vi "Calinski_Harabasz_Score.vi"(8 "error in (no error)":errorcluster caption="entrée d'erreur (pas d'erreur)", 10 "labels":string[][](array[string]), 11 "X":string[][](array[string])) -> (0 "error out":errorcluster caption="sortie d'erreur", 3 "Score":string)   [LabVIEW 2020]
doc: "Compute the Calinski and Harabasz score.\n\nIt is also known as the Variance Ratio Criterion.\n\nThe score is defined as ratio between the within-cluster dispersion and the between-cluster dispersion.\n\n\n\nParameters : \n\n- X : array-like, shape (n_samples, n_features)\nList of n_features-dimensional data points. Each row corresponds to a single data point.\n\n- labels : array-like, shape (n_samples,)\nPredicted labels for each sample.\n\nReturns : \n\n- score : float\nThe resulting Calinski-Harabasz score."
uses:
  Calinski_Harabasz_Score.lvclass
panel:
  out "Calinski_Harabasz_Score.lvclass":refnum<class "Calinski_Harabasz_Score.lvclass">
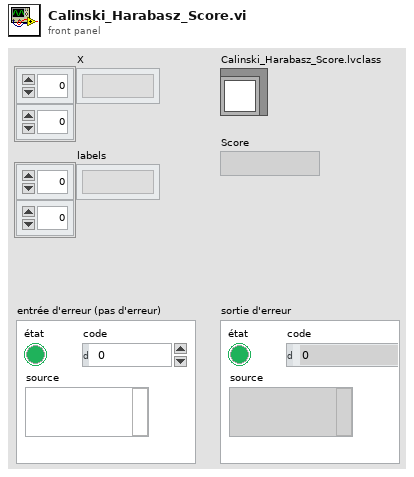
[diagram p1: front panel]
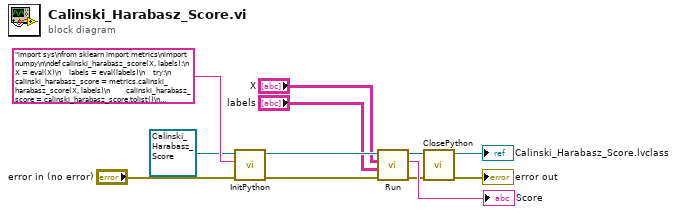
[diagram p0: block diagram]
diagram:
  n1 = call-dynamic "InitPython.vi"("error in (no error)"="error in (no error)", "Python Instruction"="import sys\nfrom sklearn import metrics\nimport numpy\n\ndef calinski_harabasz_score(X, labels):\n    X = eval(X)\n    labels = eval(labels)\n    try:\n        calinski_harabasz_score = metrics.calinski_harabasz_score(X, labels)\n        calinski_harabasz_score = calinski_harabasz_score.tolist()\n        return str(calinski_harabasz_score)\n    except:\n        erreur = sys.exc_info()\n        typerr = u\"%s\" % (erreur[0])\n        typerr = typerr[typerr.find(\"'\")+1:typerr.rfind(\"'\")]\n        msgerr = u\"%s\" % (erreur[1])\n        message = str('/!\\\\ {0} : {1}'. format(typerr,msgerr))\n        return message", "Scikit-learn en entrée"=refnum<class "Calinski_Harabasz_Score.lvclass"> refnum ("Calinski_Harabasz_Score.lvclass")) -> ("error out"=w7:errorcluster, "Scikit-learn en sortie"=w8:refnum<class "Calinski_Harabasz_Score.lvclass">)  [unwired: 7 in]
  n2 = call-dynamic "Run.vi"("error in (no error)"=w7, "labels"="labels", "X"="X", "Calinski_Harabasz_Score.lvclass"=w8) -> ("error out"=w4:errorcluster, "String Data"=→"Score":string, "Calinski_Harabasz_Score.lvclass"=w6:refnum<class "Calinski_Harabasz_Score.lvclass">)  [unwired: 5 in]
  n3 = call-dynamic "ClosePython.vi"("error in (no error)"=w4, "Scikit-learn en entrée"=w6) -> ("error out"=→"error out":errorcluster, "Scikit-learn en sortie"=→"Calinski_Harabasz_Score.lvclass":refnum<class "Calinski_Harabasz_Score.lvclass">)  [unwired: 8 in]
